vi "Close Sessions Impl.vi"(8 "error in":errorcluster, 11 "data in":T1) -> (0 "error out":errorcluster, 3 "data out":T1)   [LabVIEW 2020, in "MeasurementLink Session Management.lvlib" / "Session Reservation.lvclass"]
doc: "Closes all open sessions in the reservation."
uses:
  Session Reservation.lvclass
  Data.ctl
  Connection Map/Connection Map.lvclass
  IState/IState.lvclass
  Session and Driver Info.ctl
  MeasurementLink Instrument/IInstrument/IInstrument.lvclass
  MeasurementLink Session Management Client/RPC Messages/ni_measurementlink_sessionmanagement_v1_SessionInformation.ctl
  MeasurementLink Session Management Client/RPC Messages/nidevice_grpc_Session.ctl
  MeasurementLink Session Management Client/RPC Messages/ni_measurementlink_sessionmanagement_v1_ChannelMapping.ctl
  MeasurementLink Session Management Client/RPC Messages/ni_measurementlink_PinMapContext.ctl
  MeasurementLink Instrument/IInstrument/Close Session Behavior.ctl
  MeasurementLink Session Management Client/MeasurementLink Session Management Client.lvlib
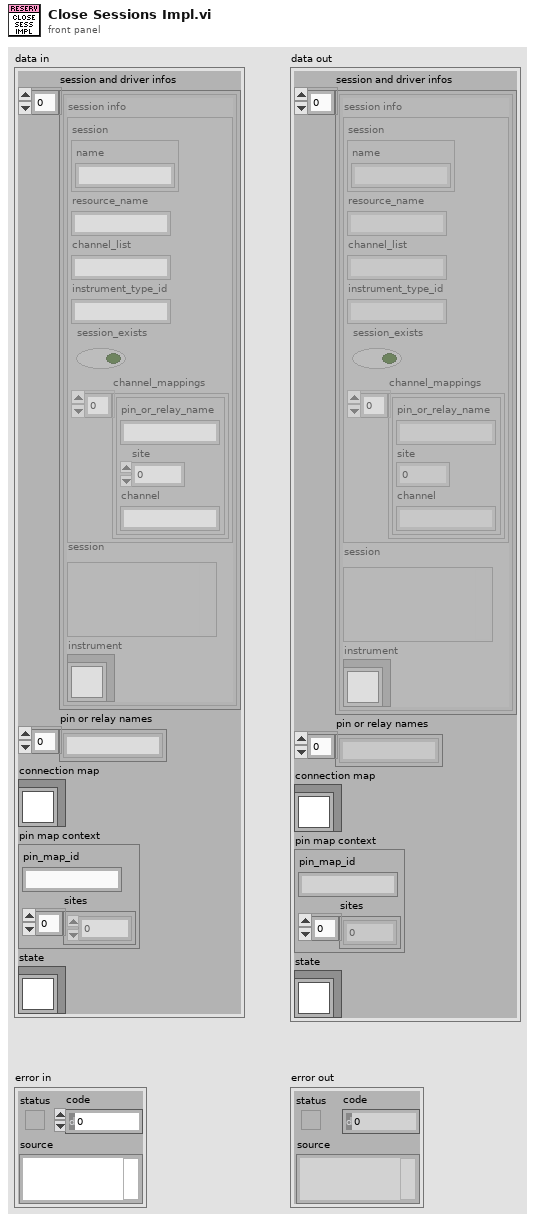
[diagram p1: front panel]
types:
  T1 = typedef "MeasurementLink Session Management.lvlib/Session Reservation.lvclass/Data.ctl" = cluster{"session and driver infos":T2[], "pin or relay names":string[], "connection map":refnum<class "Connection Map.lvclass">, "pin map context":T6, "state":refnum<class "IState.lvclass">}
  T2 = typedef "MeasurementLink Session Management.lvlib/Session Reservation.lvclass/Session and Driver Info.ctl" = cluster{"session info":T3, "session":variant, "instrument":refnum<class "IInstrument.lvclass">}
  T3 = typedef "MeasurementLink Session Management Client.lvlib/ni_measurementlink_sessionmanagement_v1_SessionInformation.ctl" = cluster{"session":T4, "resource_name":string, "channel_list":string, "instrument_type_id":string, "session_exists":bool, "channel_mappings":T5[]}
  T4 = typedef "MeasurementLink Session Management Client.lvlib/nidevice_grpc_Session.ctl" = cluster{"name":string}
  T5 = typedef "MeasurementLink Session Management Client.lvlib/ni_measurementlink_sessionmanagement_v1_ChannelMapping.ctl" = cluster{"pin_or_relay_name":string, "site":i32, "channel":string}
  T6 = typedef "MeasurementLink Session Management Client.lvlib/ni_measurementlink_PinMapContext.ctl" = cluster{"pin_map_id":string, "sites":i32[]}
  T7 = typedef "MeasurementLink Instrument.lvlib/IInstrument.lvclass/Close Session Behavior.ctl" = enum16{"Close Session", "Detach Session"}
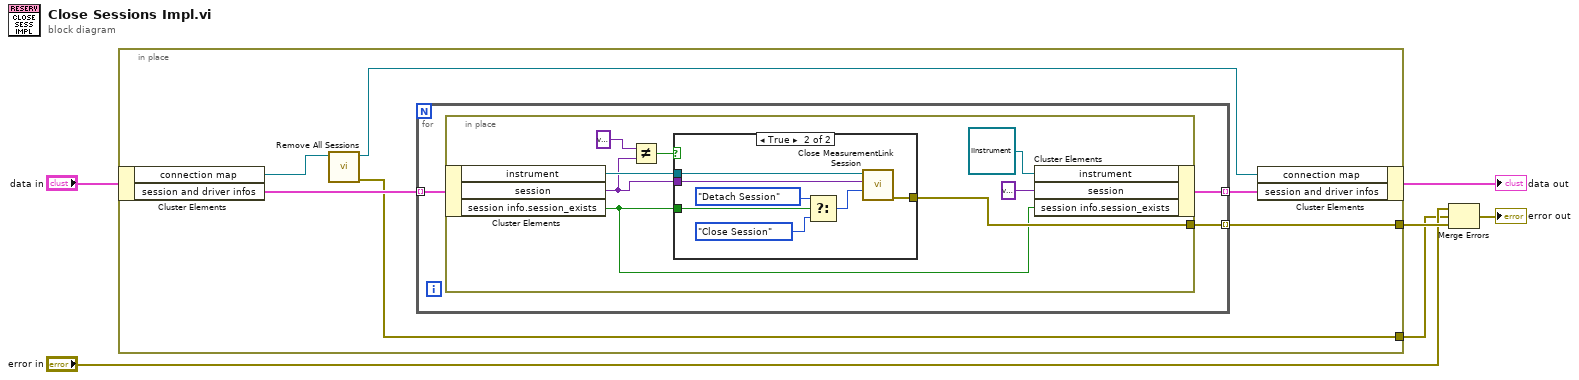
[diagram p0: block diagram]
diagram:
  n1 = in-place {
    in-place-border: [w10] -> w6
    in-place-border: [w9] -> w3
    n2 = in-place-cluster #1("data in") -> ("connection map"=w8:refnum<class "Connection Map.lvclass">, "session and driver infos"=w12:T2[])
    n3 = call "Remove All Sessions.vi"("connection map in"=w8) -> ("error out"=w9:errorcluster, "connection map out"=w7:refnum<class "Connection Map.lvclass">)  [unwired: 9 in]
    n4 = for {
      tunnel: w12 -> [w15] mode=indexing
      tunnel: [w14] -> w11 mode=indexing
      tunnel: [w13] -> w10 mode=indexing
      n5 = in-place {
        in-place-border: [w22] -> w13
        n6 = in-place-cluster #2(w15) -> ("instrument"=w21:refnum<class "IInstrument.lvclass">, "session"=w17:variant, "session info.session_exists"=w19:bool)
        n7 = Not Equal?(x=variant, y=w17) -> (x != y?=w18:bool)
        n8 = case shown="True" w18 {
          tunnel: w17 -> [_ w30]
          tunnel: [_ w29] -> w22
          tunnel: w21 -> [_ w28]
          tunnel: w19 -> [_ w24]
          frame False {
          }
          frame True {
            n9 = Select(t=Close_Session_Behavior."Detach Session" ("close session behavior"), s=w24, f=Close_Session_Behavior."Close Session" ("close session behavior")) -> (s? t:f=w25:T7)
            n10 = call-dynamic "Close MeasurementLink Session.vi"("close session behavior"=w25, "session in"=w30, "instrument in"=w28) -> ("error out"=w29:errorcluster)  [unwired: 8 in]
          }
        }
        n11 = in-place-cluster #2("instrument"=refnum<class "IInstrument.lvclass"> refnum, "session"=variant, "session info.session_exists"=w19) -> (w14:T2)
      }
    }
    n12 = in-place-cluster #1("connection map"=w7, "session and driver infos"=w11) -> (→"data out":T1)
  }
  n13 = Merge Errors("error in", w3, w6) -> (→"error out":errorcluster)
